vi "Init Teller.vi"(9 "Relation":T1, 10 "Self Attributes":refnum<class "Attributes.lvclass">) -> (3 "Base Teller out":refnum<class "Base Teller.lvclass">)   [LabVIEW 2025, in "jettl.lvlib" / "Teller.lvlib" / "Base Teller.lvclass"]
uses:
  Base Teller.lvclass
  Relation.ctl
  Attributes/Attributes/Attributes.lvclass
  Base Teller.lvclass/Base Teller.ctl
  jettl.lvlib
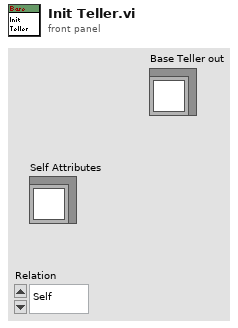
[diagram p1: front panel]
types:
  T1 = typedef "jettl.lvlib/Relation.ctl" = enum16{"Self", "Parent", "Child"}
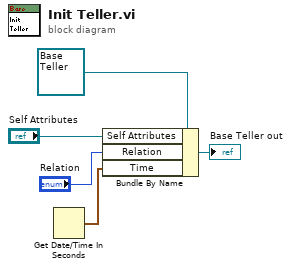
[diagram p0: block diagram]
diagram:
  n1 = Get Date/Time In Seconds() -> (seconds since 1Jan1904=w3:timestamp)
  n2 = Bundle By Name(cluster=refnum<class "Base Teller.lvclass"> refnum ("Base Sender out"), "Self Attributes"="Self Attributes", "Relation"="Relation", "Time"=w3) -> (→"Base Teller out":refnum<class "Base Teller.lvclass">)
